vi "Concatenate Topologies.vi"(9 "Topology B":T1, 11 "Topology A":T1) -> (2 "Concatenated":T1)   [LabVIEW 2016, in "SLSC Switch.lvlib" / "SLSC Switch.lvclass"]
uses:
  SLSC Switch.lvclass
  Controls/Topology.ctl
  Controls/JSON.InitialState.ctl
  Controls/JSON.ChannelList.ctl
  Controls/JSON.ConnectionList.ctl
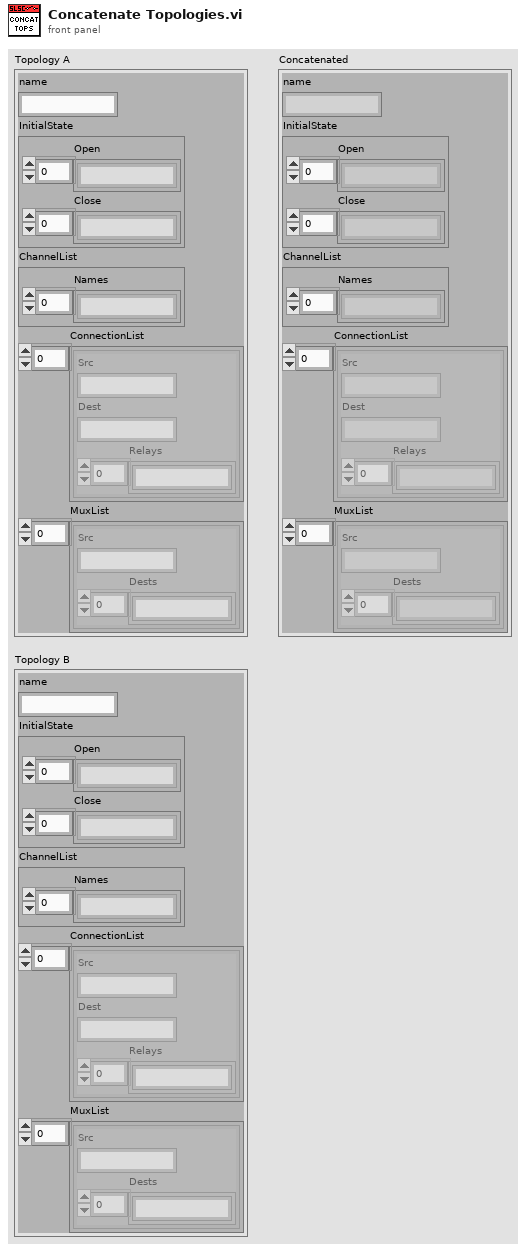
[diagram p1: front panel]
types:
  T1 = typedef "SLSC Switch.lvlib/SLSC Switch.lvclass/Topology.ctl" = cluster{"name":string, "InitialState":T2, "ChannelList":T3, "ConnectionList":T4[], "MuxList":cluster{"Src":string, "Dests":string[]}[]}
  T2 = typedef "SLSC Switch.lvlib/SLSC Switch.lvclass/JSON.InitialState.ctl" = cluster{"Open":string[], "Close":string[]}
  T3 = typedef "SLSC Switch.lvlib/SLSC Switch.lvclass/JSON.ChannelList.ctl" = cluster{"Names":string[]}
  T4 = typedef "SLSC Switch.lvlib/SLSC Switch.lvclass/JSON.ConnectionList.ctl" = cluster{"Src":string, "Dest":string, "Relays":string[]}
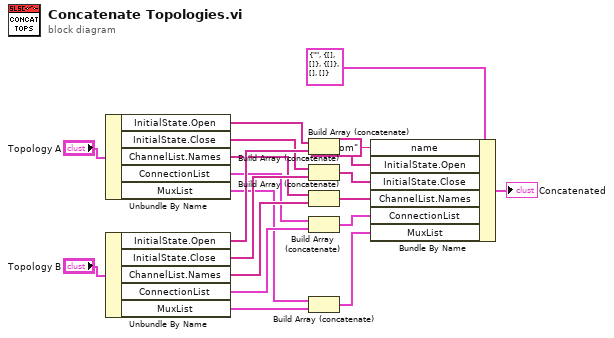
[diagram p0: block diagram]
diagram:
  n1 = Unbundle By Name("Topology A") -> ("InitialState.Open"=w18:string[], "InitialState.Close"=w16:string[], "ChannelList.Names"=w14:string[], "ConnectionList"=w12:T4[], "MuxList"=w10:cluster{"Src":string, "Dests":string[]}[])
  n2 = Unbundle By Name("Topology B") -> ("InitialState.Open"=w17:string[], "InitialState.Close"=w15:string[], "ChannelList.Names"=w13:string[], "ConnectionList"=w11:T4[], "MuxList"=w9:cluster{"Src":string, "Dests":string[]}[])
  n3 = Build Array (concatenate)(w18, w17) -> (w7:string[])
  n4 = Build Array (concatenate)(w16, w15) -> (w6:string[])
  n5 = Build Array (concatenate)(w14, w13) -> (w5:string[])
  n6 = Build Array (concatenate)(w12, w11) -> (w4:T4[])
  n7 = Build Array (concatenate)(w10, w9) -> (w3:cluster{"Src":string, "Dests":string[]}[])
  n8 = Bundle By Name(cluster=T1 {"name"="", "InitialState"={"Open"=[], "Close"=[]}, "ChannelList"={"Names"=[]}, "ConnectionList"=[], "MuxList"=[]} ("Topology A"), "name"="Custom", "InitialState.Open"=w7, "InitialState.Close"=w6, "ChannelList.Names"=w5, "ConnectionList"=w4, "MuxList"=w3) -> (→"Concatenated":T1)
